vi "Get Image Delays.vi"(8 "error in (no error)":errorcluster, 10 "frames":u16, 11 "Simulated_Header in":refnum<class "Simulated_Header.lvclass">) -> (0 "error out":errorcluster, 3 "Simulated_Header out":refnum<class "Simulated_Header.lvclass">)   [LabVIEW 2018, in "Simulated_Header.lvclass"]
uses:
  Simulated_Header.lvclass
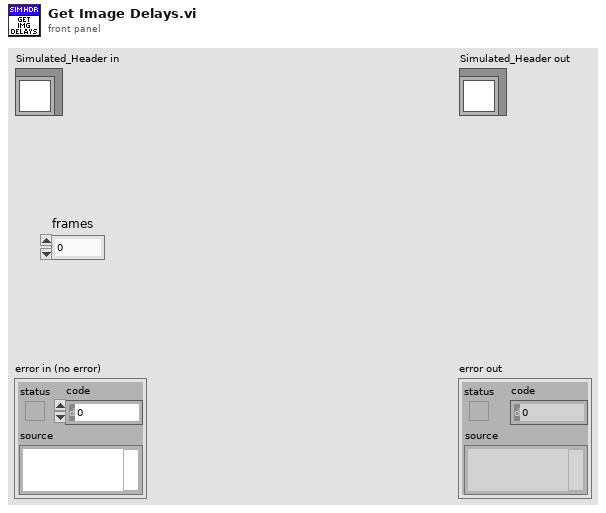
[diagram p1: front panel]
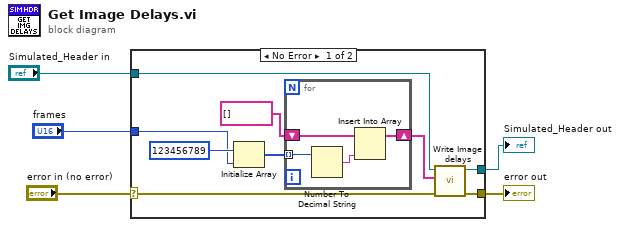
[diagram p0: block diagram]
diagram:
  n1 = case shown="No Error" "error in (no error)" {
    selector: "error in (no error)" -> [w9 w20]
    tunnel: [w7 w20] -> w3
    tunnel: [w8 w19] -> w2
    tunnel: "Simulated_Header in" -> [w10 w19]
    tunnel: "frames" -> [w6 _]
    frame No Error {
      n2 = Initialize Array(123456789, w6) -> (w12:i32[])
      n3 = for {
        shift-right: [w15] -> w11
        shift-left: string[] [] -> [w16]
        tunnel: w12 -> [w18] mode=indexing
        n4 = Number To Decimal String(number=w18) -> (decimal integer string=w17:string)  [unwired: 1 in]
        n5 = Insert Into Array(array=w16, new element=w17) -> (w15:string[])  [unwired: 1 in]
      }
      n6 = call "Write Image delays.vi"("error in (no error)"=w9, "Image delays"=w11, "Header in"=w10) -> ("error out"=w7:errorcluster, "Header out"=w8:refnum<class "Simulated_Header.lvclass">)  [unwired: 7 in]
    }
    frame Error {
    }
  }
  "error out" <- w3
  "Simulated_Header out" <- w2
